vi "Get Thread Configuration.vi"(8 "error in (no error)":errorcluster, 11 "Component Configuration in":refnum<class "PXImc Configurations.lvclass">) -> (0 "error out":errorcluster, 2 "Thread Configuration":refnum<class "Configuration.lvclass">, 3 "Component Configuration out":refnum<class "PXImc Configurations.lvclass">)   [LabVIEW 2017, in "PXImc.lvlib" / "PXImc Configurations.lvclass"]
uses:
  PXImc Configurations.lvclass
  DSF Core.lvlibp/Classes/Configuration/Configuration.lvclass
  Thread/Thread Configuration.lvclass
  C:/Git/DSF/Components/DSF Core.lvlibp/Classes/Configuration/Configuration.lvclass
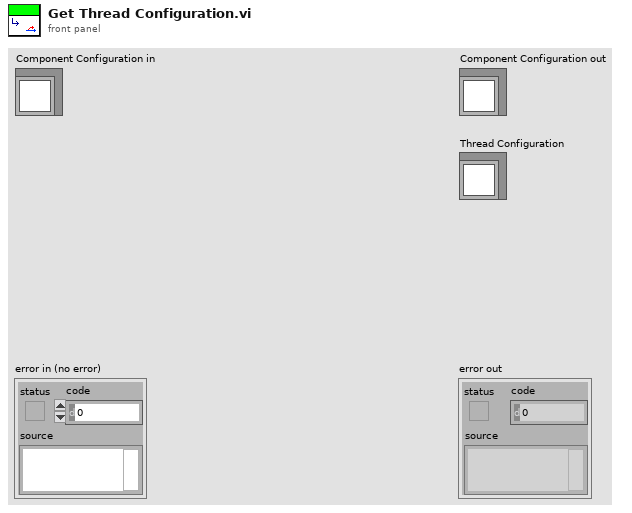
[diagram p1: front panel]
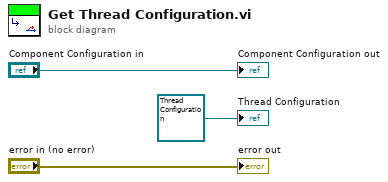
[diagram p0: block diagram]
diagram:
  "error out" <- "error in (no error)"
  "Component Configuration out" <- "Component Configuration in"
  "Thread Configuration" <- refnum<class "Thread Configuration.lvclass"> refnum ("PXImc.lvlib:PXImc Thread Configuration")
